vi "Element Type.vi"(11 "DblNumericStatusIndicator in":refnum<class "DblNumericStatusIndicator.lvclass">) -> (2 "Indicator Type":string)   [LabVIEW 2020, in "VolatusGUIElements.lvlib" / "DblNumericStatusIndicator.lvclass"]
uses:
  DblNumericStatusIndicator.lvclass
  DblNumericStatusIndicator.lvclass/DblNumericStatusIndicator.ctl
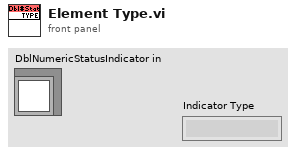
[diagram p1: front panel]
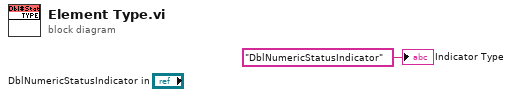
[diagram p0: block diagram]
diagram:
  "Indicator Type" <- "DblNumericStatusIndicator" ("Indicator Type")
